vi "5.10 Filter Control Math.vi"(1 "Gains and Parameters":T1={"Control Gain"=0.0, "Line Setpoint in Pixels"=0.0, "Low Pass Gain"=0.0, "Image Low Pass Gain"=0.0, "Line Fullness Setpoint"=0.0, "Line Fullness Std"=0.1, "Max Filter Mod"=-10.0}, 2 "Lower Std Deviation":dbl, 3 "Fullness":dbl) -> (0 "Control Output":dbl)   [LabVIEW 2010]
uses:
  5.10 Algorithm Parameters and Controls.ctl
  <vilib>/gmath/statdist.llb/Normal PDF.vi
  <vilib>/gmath/NI_Gmath.lvlib
panel:
  in  "A reasonable fullness for a line":dbl=0.1
  in  "std":dbl=0.1
  out "pdf(x)":dbl=0.3989422804014327
  out "Line Width Behavior":dbl[](array[numeric])
  out "Fullness behavior":dbl[](array[numeric])
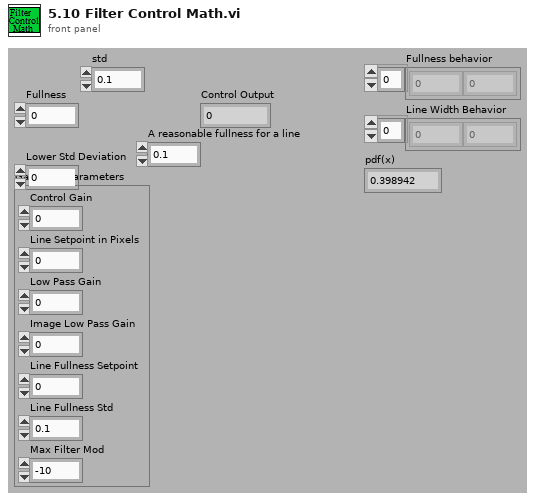
[diagram p1: front panel]
types:
  T1 = typedef "5.10 Algorithm Parameters and Controls.ctl" = cluster{"Control Gain":dbl, "Line Setpoint in Pixels":dbl, "Low Pass Gain":dbl, "Image Low Pass Gain":dbl, "Line Fullness Setpoint":dbl, "Line Fullness Std":dbl, "Max Filter Mod":dbl}
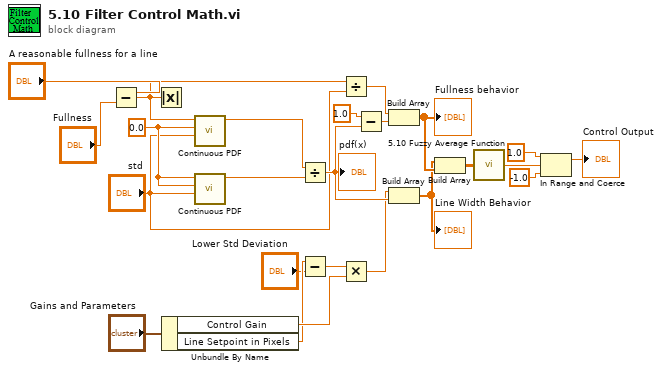
[diagram p0: block diagram]
diagram:
  w8 = 0.0 ("mean")
  n1 = Subtract(x="A reasonable fullness for a line", y="Fullness") -> (x-y=w3:dbl)
  n2 = Absolute Value(x=w3) -> ()  [unwired: 1 out]
  n3 = Unbundle By Name("Gains and Parameters") -> ("Control Gain"=w18:dbl, "Line Setpoint in Pixels"=w13:dbl)
  n4 = call-poly <vilib>:"Continuous PDF.vi"("std"="std", "mean"=w8, "x"=w3) -> ("pdf(x)"=w16:dbl)  [unwired: 7 in, 1 out]
  n5 = call-poly <vilib>:"Continuous PDF.vi"("std"="std", "mean"=w8, "x"=w8) -> ("pdf(x)"=w6:dbl)  [unwired: 7 in, 1 out]
  n6 = Divide(x=w16, y=w6) -> (x/y=w7:dbl)
  "pdf(x)" <- w7
  n7 = Subtract(x=w13, y="Lower Std Deviation") -> (x-y=w4:dbl)
  n8 = Divide(x=w3, y="std") -> (x/y=w2:dbl)
  n9 = Multiply(x=w4, y=w18) -> (x*y=w5:dbl)
  n10 = Subtract(x=1.0, y=w7) -> (x-y=w17:dbl)
  n11 = Build Array(w2, w17) -> (w20:dbl[])
  "Fullness behavior" <- w20
  n12 = Build Array(w5, w7) -> (w19:dbl[])
  "Line Width Behavior" <- w19
  n13 = Build Array(w19, w20) -> (w21:dbl[][])
  n14 = call "5.10 Fuzzy Average Function.vi"("Input Control Certainty Array"=w21) -> ("Output Control Value"=w22:dbl)
  n15 = In Range and Coerce(upper limit=1.0, x=w22, lower limit=-1.0 ("upper limit")) -> (coerced(x)=→"Control Output":dbl)  [unwired: 1 out]
